vi "test--ui.vi"() -> ()   [LabVIEW 2021]
doc: "This VI will be used to test out the label creation and deletion, the quick drop list of controls, and the theme change"
panel:
  in  "String":string
  in  "filled--text--rectangular":bool
  in  "tonal--icons--rounded":bool
  in  "outline--text--rectangular":bool
  in  "FAB Button":bool
  out "header":bool
  # "Free Label"
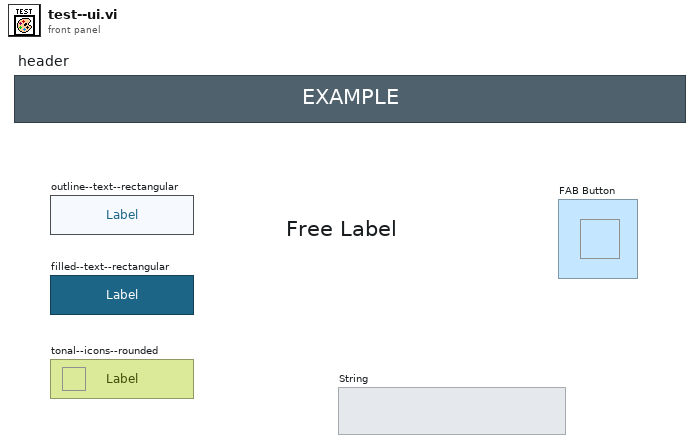
[diagram p1: front panel]
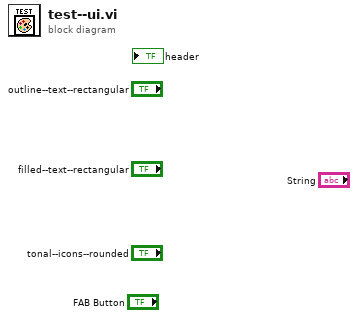
[diagram p0: block diagram]
diagram:
